vi "Enqueue Message (Multiple).vi"(6 "Priority Message?":bool[](array[boolean]), 8 "error in (no error)":errorcluster, 9 "Data":variant[](array[variant]), 10 "States":i32[](array[numeric]), 11 "Message Queue in":refnum<queue>) -> (0 "error out":errorcluster, 3 "Message Queue out":refnum<queue>)   [LabVIEW 2016, in "Message Queue.lvlib"]
uses:
  Message Queue.lvlib
  Message.ctl
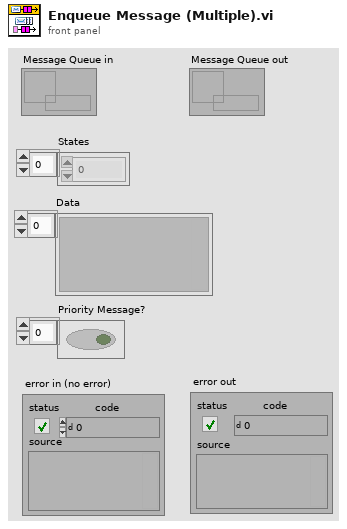
[diagram p1: front panel]
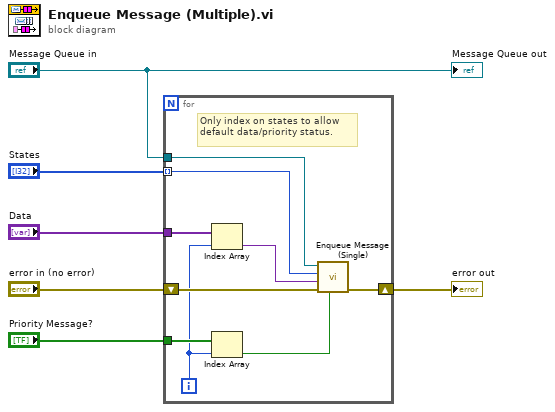
[diagram p0: block diagram]
diagram:
  n1 = for {
    shift-right: [w14] -> w5
    shift-left: "error in (no error)" -> [w15]
    tunnel: "Message Queue in" -> [w13]
    tunnel: "States" -> [w12] mode=indexing
    tunnel: "Data" -> [w11]
    tunnel: "Priority Message?" -> [w10]
    i -> [w9]
    # "Only index on states to allow default data/priority status."
    n2 = Index Array(array=w11, index=w9) -> (element=w8:variant)
    n3 = Index Array(array=w10, index=w9) -> (element=w7:bool)
    n4 = call "Enqueue Message (Single).vi"("High Priority?"=w7, "error in (no error)"=w15, "Data"=w8, "State"=w12, "Message Queue in"=w13) -> ("error out"=w14:errorcluster)  [unwired: 5 in, 1 out]
  }
  "error out" <- w5
  "Message Queue out" <- "Message Queue in"
